vi "HEWH First Hour Rating Previous Terminate Value.vi"(8 "Error In":errorcluster, 11 "FileInit Cluster":T1={"Scan Rate Adjust"=0.0, "Draw Count"=0, "Test Patten Setup"={"Total Gallons Schedule"=[], "PRAT/RLT Sequence"=[{"Sequence #"=1.0, "Cycles"=35, "Mode Setting"="", "Flow Rate (GPM)"=0.0, "Temperature (F)"=0.0, "Reset Timer"=FALSE, "Use Temp Decline Method"=FALSE, "Terminate Condition"=enum."C1-Terminate Draw @ Gallon Mark", "Condition Value #1"=0.0, "UE"=FALSE, "LE"=FALSE, "Comp"=FALSE, "Fan"=FALSE, "Test End Time (Sec)"=0.0, "Purge Until Cutout"=FALSE, "Start Conditions"=enum."Heat Source Cutout", "Condition Value #2"=0.0, "Remove Power"=FALSE, "Time"=0.0, "Check Special Cond."=enum."SC1-Do Nothing", "Condition#"=enum."C1", "Draw Flags"=enum."N/A", "Data Processing Delay (FHD 15sec, UEF 5 Sec)"=0.0, "Test Complete"=FALSE}, {"Sequence #"=2.0, "Cycles"=15, "Mode Setting"="", "Flow Rate (GPM)"=0.0, "Temperature (F)"=0.0, "Reset Timer"=FALSE, "Use Temp Decline Method"=FALSE, "Terminate Condition"=enum."C1-Terminate Draw @ Gallon Mark", "Condition Value #1"=0.0, "UE"=FALSE, "LE"=FALSE, "Comp"=FALSE, "Fan"=FALSE, "Test End Time (Sec)"=0.0, "Purge Until Cutout"=FALSE, "Start Conditions"=enum."Heat Source Cutout", "Condition Value #2"=0.0, "Remove Power"=FALSE, "Time"=0.0, "Check Special Cond."=enum."SC1-Do Nothing", "Condition#"=enum."C1", "Draw Flags"=enum."N/A", "Data Processing Delay (FHD 15sec, UEF 5 Sec)"=0.0, "Test Complete"=FALSE}, {"Sequence #"=3.0, "Cycles"=35, "Mode Setting"="", "Flow Rate (GPM)"=0.0, "Temperature (F)"=0.0, "Reset Timer"=FALSE, "Use Temp Decline Method"=FALSE, "Terminate Condition"=enum."C1-Terminate Draw @ Gallon Mark", "Condition Value #1"=0.0, "UE"=FALSE, "LE"=FALSE, "Comp"=FALSE, "Fan"=FALSE, "Test End Time (Sec)"=0.0, "Purge Until Cutout"=FALSE, "Start Conditions"=enum."Heat Source Cutout", "Condition Value #2"=0.0, "Remove Power"=FALSE, "Time"=0.0, "Check Special Cond."=enum."SC1-Do Nothing", "Condition#"=enum."C1", "Draw Flags"=enum."N/A", "Data Processing Delay (FHD 15sec, UEF 5 Sec)"=0.0, "Test Complete"=FALSE}, {"Sequence #"=4.0, "Cycles"=15, "Mode Setting"="", "Flow Rate (GPM)"=0.0, "Temperature (F)"=0.0, "Reset Timer"=FALSE, "Use Temp Decline Method"=FALSE, "Terminate Condition"=enum."C1-Terminate Draw @ Gallon Mark", "Condition Value #1"=0.0, "UE"=FALSE, "LE"=FALSE, "Comp"=FALSE, "Fan"=FALSE, "Test End Time (Sec)"=0.0, "Purge Until Cutout"=FALSE, "Start Conditions"=enum."Heat Source Cutout", "Condition Value #2"=0.0, "Remove Power"=FALSE, "Time"=0.0, "Check Special Cond."=enum."SC1-Do Nothing", "Condition#"=enum."C1", "Draw Flags"=enum."N/A", "Data Processing Delay (FHD 15sec, UEF 5 Sec)"=0.0, "Test Complete"=FALSE}, {"Sequence #"=5.0, "Cycles"=35, "Mode Setting"="", "Flow Rate (GPM)"=0.0, "Temperature (F)"=0.0, "Reset Timer"=FALSE, "Use Temp Decline Method"=FALSE, "Terminate Condition"=enum."C1-Terminate Draw @ Gallon Mark", "Condition Value #1"=0.0, "UE"=FALSE, "LE"=FALSE, "Comp"=FALSE, "Fan"=FALSE, "Test End Time (Sec)"=0.0, "Purge Until Cutout"=FALSE, "Start Conditions"=enum."Heat Source Cutout", "Condition Value #2"=0.0, "Remove Power"=FALSE, "Time"=0.0, "Check Special Cond."=enum."SC1-Do Nothing", "Condition#"=enum."C1", "Draw Flags"=enum."N/A", "Data Processing Delay (FHD 15sec, UEF 5 Sec)"=0.0, "Test Complete"=FALSE}, {"Sequence #"=6.0, "Cycles"=15, "Mode Setting"="", "Flow Rate (GPM)"=0.0, "Temperature (F)"=0.0, "Reset Timer"=FALSE, "Use Temp Decline Method"=FALSE, "Terminate Condition"=enum."C1-Terminate Draw @ Gallon Mark", "Condition Value #1"=0.0, "UE"=FALSE, "LE"=FALSE, "Comp"=FALSE, "Fan"=FALSE, "Test End Time (Sec)"=0.0, "Purge Until Cutout"=FALSE, "Start Conditions"=enum."Heat Source Cutout", "Condition Value #2"=0.0, "Remove Power"=FALSE, "Time"=0.0, "Check Special Cond."=enum."SC1-Do Nothing", "Condition#"=enum."C1", "Draw Flags"=enum."N/A", "Data Processing Delay (FHD 15sec, UEF 5 Sec)"=0.0, "Test Complete"=FALSE}, {"Sequence #"=7.0, "Cycles"=35, "Mode Setting"="", "Flow Rate (GPM)"=0.0, "Temperature (F)"=0.0, "Reset Timer"=FALSE, "Use Temp Decline Method"=FALSE, "Terminate Condition"=enum."C1-Terminate Draw @ Gallon Mark", "Condition Value #1"=0.0, "UE"=FALSE, "LE"=FALSE, "Comp"=FALSE, "Fan"=FALSE, "Test End Time (Sec)"=0.0, "Purge Until Cutout"=FALSE, "Start Conditions"=enum."Heat Source Cutout", "Condition Value #2"=0.0, "Remove Power"=FALSE, "Time"=0.0, "Check Special Cond."=enum."SC1-Do Nothing", "Condition#"=enum."C1", "Draw Flags"=enum."N/A", "Data Processing Delay (FHD 15sec, UEF 5 Sec)"=0.0, "Test Complete"=FALSE}, {"Sequence #"=8.0, "Cycles"=15, "Mode Setting"="", "Flow Rate (GPM)"=0.0, "Temperature (F)"=0.0, "Reset Timer"=FALSE, "Use Temp Decline Method"=FALSE, "Terminate Condition"=enum."C1-Terminate Draw @ Gallon Mark", "Condition Value #1"=0.0, "UE"=FALSE, "LE"=FALSE, "Comp"=FALSE, "Fan"=FALSE, "Test End Time (Sec)"=0.0, "Purge Until Cutout"=FALSE, "Start Conditions"=enum."Heat Source Cutout", "Condition Value #2"=0.0, "Remove Power"=FALSE, "Time"=0.0, "Check Special Cond."=enum."SC1-Do Nothing", "Condition#"=enum."C1", "Draw Flags"=enum."N/A", "Data Processing Delay (FHD 15sec, UEF 5 Sec)"=0.0, "Test Complete"=FALSE}], "Current Sequence Index"=0}, "HEWH Specific DAQ"={"HEWH Data"={"HEWH Standard"={"Voltage (Volts)"=0.0, "Current (Amps)"=0.0, "Power (Watts)"=0.0, "WattHours (Wh)"=0.0, "TC Tree (AVG)"=0.0, "Flow Rate (GPM)"=0.0, "Gallons (Gal)"=0.0, "RTD Out (Deg F)"=0.0, "RTD In (Deg F)"=0.0, "RTD Amb (Deg F)"=0.0, "TC Down"=0.0, "UE Event Lead"=0, "LE Event Lead"=0, "TC Tree Array"=[]}, "PRAT"={"Power (Watts) A"=4192.0, "Power (Watts) B"=4192.0, "Power (Watts) C"=4192.0, "Power (Watts) D"=4192.0, "TC1"=0.0, "TC2"=0.0, "TC3"=0.0, "TC4"=0.0, "WattHours (Wh) A"=4192.0, "WattHours (Wh) B"=4192.0, "WattHours (Wh) C"=4192.0, "WattHours (Wh) D"=4192.0, "Ambient"=0.0, "Extra Temp"=0.0}, "Additional Power Data"={"Vthd"=236.2, "Frequency (Hz)"=236.2, "Apparent Power (VA)"=236.2, "Power Factor"=236.2, "Current Crest Factor"=236.2, "Voltage Crest Factor"=236.2, "Integration Time (sec)"=236.2}}, "Flow Valve % Open"=0.0, "Power State"={"UE"=FALSE, "LE"=FALSE, "COMP"=FALSE, "FANS"=FALSE}, "Power Analyzer"=enum."", "Flow Valve uA Output"=0, "Gallons Start (Gal)"=0.0}, "Test Output Data"={"PreDraw Data Table"=[], "Data Table"=[], "MW100 TC Headers"=[]}, "Calc and Calibration"={"Mean SD Var Max Min Array"=[], "Draw Statistics (DBL)"=[], "Calibration Coefficients DBL"=[], "Start Gallons"=0.0, "Starting Temp Decline"=0.0, "K-Factor (Intellifaucet)"=0.0, "All Draw Stats"=[], "RTD Terminate Value"=0.0}, "Current Draw Time"=0.0, "LV Program"=enum."HEWH", "Station ID"=enum."A", "Current Cond"=enum."N/A", "Test Complete"=FALSE} {"Test Patten Setup"."PRAT/RLT Sequence"."Time" format="%<%H:%M:%S>t"; "Test Patten Setup"."Total Gallons Schedule" format="%.2f"}) -> (0 "Error Out":errorcluster, 3 "Previous Terminate Value":dbl=115.0)   [LabVIEW 2016]
uses:
  Type Definitions/HEWH Output Information.ctl
  Type Definitions/HEWH Draw Pattern Setup.ctl
  Type Definitions/PRAT Test.ctl
  Utility/Save File/File Setup (Public)/Type Definition/Save File HEWH Heating Control Mode.ctl
  Draw Water Specific/Type Definitions/Terminate Draw Conditions.ctl
  Type Definitions/HEWH Start Conditions.ctl
  Draw Water Specific/Type Definitions/Check Special Condtions.ctl
  Draw Water Specific/Type Definitions/HEWH Special Condition Check.ctl
  Type Definitions/HEWH Draw Flag ENUM.ctl
  Type Definitions/HEWH Specific DAQ.ctl
  Type Definitions/HEWH Power Data.ctl
  Type Definitions/HEWH Power Elements.ctl
  Utility/Type Definitions/UTILITY Power Analyzer.ctl
  Type Definitions/HEWH Calc and Calibration.ctl
  Utility/Save File/File Setup (Public)/Type Definition/Save File DOE LabView Program.ctl
  Custom Instrument Control/MW100/Type Definitions/Station ID Selector.ctl
  <vilib>/Utility/file.llb/Read From Spreadsheet File (string).vi
  Utility/Save File/File Setup.lvlib
panel:
  out "all rows":string[][](array[string])
  in  "file path (dialog if empty)":path
  in  "Debug":string[][](array[string])=[["Voltage (Volts) - Mean", "Voltage (Volts) - Standard Deviation", "Voltage (Volts) - Variance", "Voltage (Volts) - Max", "Voltage (Volts) - Min", "Current (Amps) - Mean", "Current (Amps) - Standard Deviation", "Current (Amps) - Variance", "Current (Amps) - Max", "Current (Amps) - Min", "Power (Watts) - Mean", "Power (Watts) - Standard Deviation", "Power (Watts) - Variance", "Power (Watts) - Max", "Power (Watts) - Min", "WattHours - Max", "WattHours - Min", "TC Tree (AVG) - Mean", "TC Tree (AVG) - Standard Deviation", "TC Tree (AVG) - Variance", "TC Tree (AVG) - Max", "TC Tree (AVG) - Min", "Flow Rate (GPM) - Mean", "Flow Rate (GPM) - Standard Deviation", "Flow Rate (GPM) - Variance", "Flow Rate (GPM) - Max", "Flow Rate (GPM) - Min", "Gallons (Gal) - Max", "Gallons (Gal) - Min", "RTD Out (°F) - Mean", "RTD Out (°F) - Standard Deviation", "RTD Out (°F) - Variance", "RTD Out (°F) - Max", "RTD Out (°F) - Min", "RTD In (°F) - Mean", "RTD In (°F) - Standard Deviation", "RTD In (°F) - Variance", "RTD In (°F) - Max", "RTD In (°F) - Min", "RTD Ambinet (°F) - Mean", "RTD Ambient (°F) - Standard Deviation", "RTD Ambinent (°F) - Variance", "RTD Ambinent (°F) - Max", "RTD Ambinent (°F) - Min", "TC Down (°F) - Mean", "TC Down (°F) - Standard Deviation", "TC Down (°F) - Variance", "TC Down (°F) - Max", "TC Down (°F) - Min", "TC1 (°F) - Mean", "TC1 (°F) - Standard Deviation", "TC1 (°F) - Variance", "TC1 (°F) - Max", "TC1 (°F) - Min", "TC2 (°F) - Mean", "TC2 (°F) - Standard Deviation", "TC2 (°F) - Variance", "TC2 (°F) - Max", "TC2 (°F) - Min", "TC3 (°F) - Mean", "TC3 (°F) - Standard Deviation", "TC3 (°F) - Variance", "TC3 (°F) - Max", "TC3 (°F) - Min", "TC4 (°F) - Mean", "TC4 (°F) - Standard Deviation", "TC4 (°F) - Variance", "TC4 (°F) - Max", "TC4 (°F) - Min", "TC5 (°F) - Mean", "TC5 (°F) - Standard Deviation", "TC5 (°F) - Variance", "TC5 (°F) - Max", "TC5 (°F) - Min", "TC6 (°F) - Mean", "TC6 (°F) - Standard Deviation", "TC6 (°F) - Variance", "TC6 (°F) - Max", "TC6 (°F) - Min", "Total Harmonic Distortion (%V) - Max", "Total Harmonic Distortion (%V) - Min", "Frequency (Hz) - Mean ", "Frequency (Hz) - Standard Deviation", "Frequency (Hz) - Variance", "Frequency (Hz) - Max", "Frequency (Hz) - Min", "Apparent Power (VA) - Mean", "Apparent Power (VA) - Standard Deviation", "Apparent Power (VA) - Variance", "Apparent Power (VA) - Max", "Apparent Power (VA) - Min", "Power Factor - Max", "Power Factor - Min", "Current Crest Factor - Max", "Current Crest Factor - Min", "Voltage Crest Factor - Max", "Voltage Crest Factor - Min", "Elapsed Time (Sec) - Max", "Elapsed Time (Sec) - Min", "Condition Value #1", "Draw Count", ""], ["240.015", "0.427", "0.183", "240.270", "238.890", "0.378", "0.815", "0.665", "2.251", "0.014", "73.509", "164.034", "26907.243", "441.200", "1.055", "0.419", "0.077", "125.490", "0.253", "0.064", "125.800", "124.917", "3.018", "0.064", "0.004", "3.160", "2.900", "1.550", "0.830", "127.000", "0.000", "0.000", "127.000", "127.000", "57.575", "0.464", "0.215", "58.700", "57.000", "70.067", "0.048", "0.002", "70.100", "70.000", "57.929", "0.524", "0.274", "58.700", "57.200", "128.500", "0.000", "0.000", "128.500", "128.500", "128.312", "0.034", "0.001", "128.400", "128.300", "128.100", "0.000", "0.000", "128.100", "128.100", "127.700", "0.000", "0.000", "127.700", "127.700", "125.454", "1.114", "1.241", "126.200", "122.700", "114.875", "0.523", "0.273", "116.000", "114.200", "1.734", "1.563", "60.025", "0.015", "0.000", "60.063", "59.998", "90.320", "194.990", "38021.086", "539.800", "3.467", "0.856", "0.296", "9.576", "1.605", "1.449", "1.418", "29.823", "15.517", "0.000", "0.000", ""], ["239.536", "0.610", "0.372", "242.500", "238.460", "7.472", "8.359", "69.877", "18.776", "0.014", "1762.908", "2029.049", "4117040.569", "4510.000", "1.035", "597.580", "255.570", "104.807", "13.752", "189.114", "128.500", "82.400", "3.003", "0.059", "0.004", "3.170", "2.800", "33.840", "0.780", "127.270", "3.423", "11.719", "131.000", "116.000", "57.578", "0.360", "0.130", "58.900", "56.800", "69.441", "0.264", "0.070", "69.900", "68.800", "57.952", "0.451", "0.203", "59.200", "56.800", "126.863", "5.421", "29.387", "131.700", "105.800", "119.154", "17.250", "297.576", "131.600", "81.000", "107.909", "22.756", "517.820", "131.500", "78.000", "96.487", "20.170", "406.839", "130.600", "77.100", "89.568", "13.478", "181.656", "127.900", "75.200", "88.858", "12.000", "144.005", "117.700", "75.400", "1.682", "1.491", "59.995", "0.014", "0.000", "60.061", "59.946", "1794.387", "2009.288", "4037238.121", "4510.000", "3.430", "1.000", "0.291", "9.827", "1.421", "1.438", "1.418", "675.733", "15.038", "15.000", "0.000", ""]]
  in  "RTD Max Min Array":string[][](array[string])=[["", "", "", ""]]
  # "Draw Pattern Setup (24 Hour)"
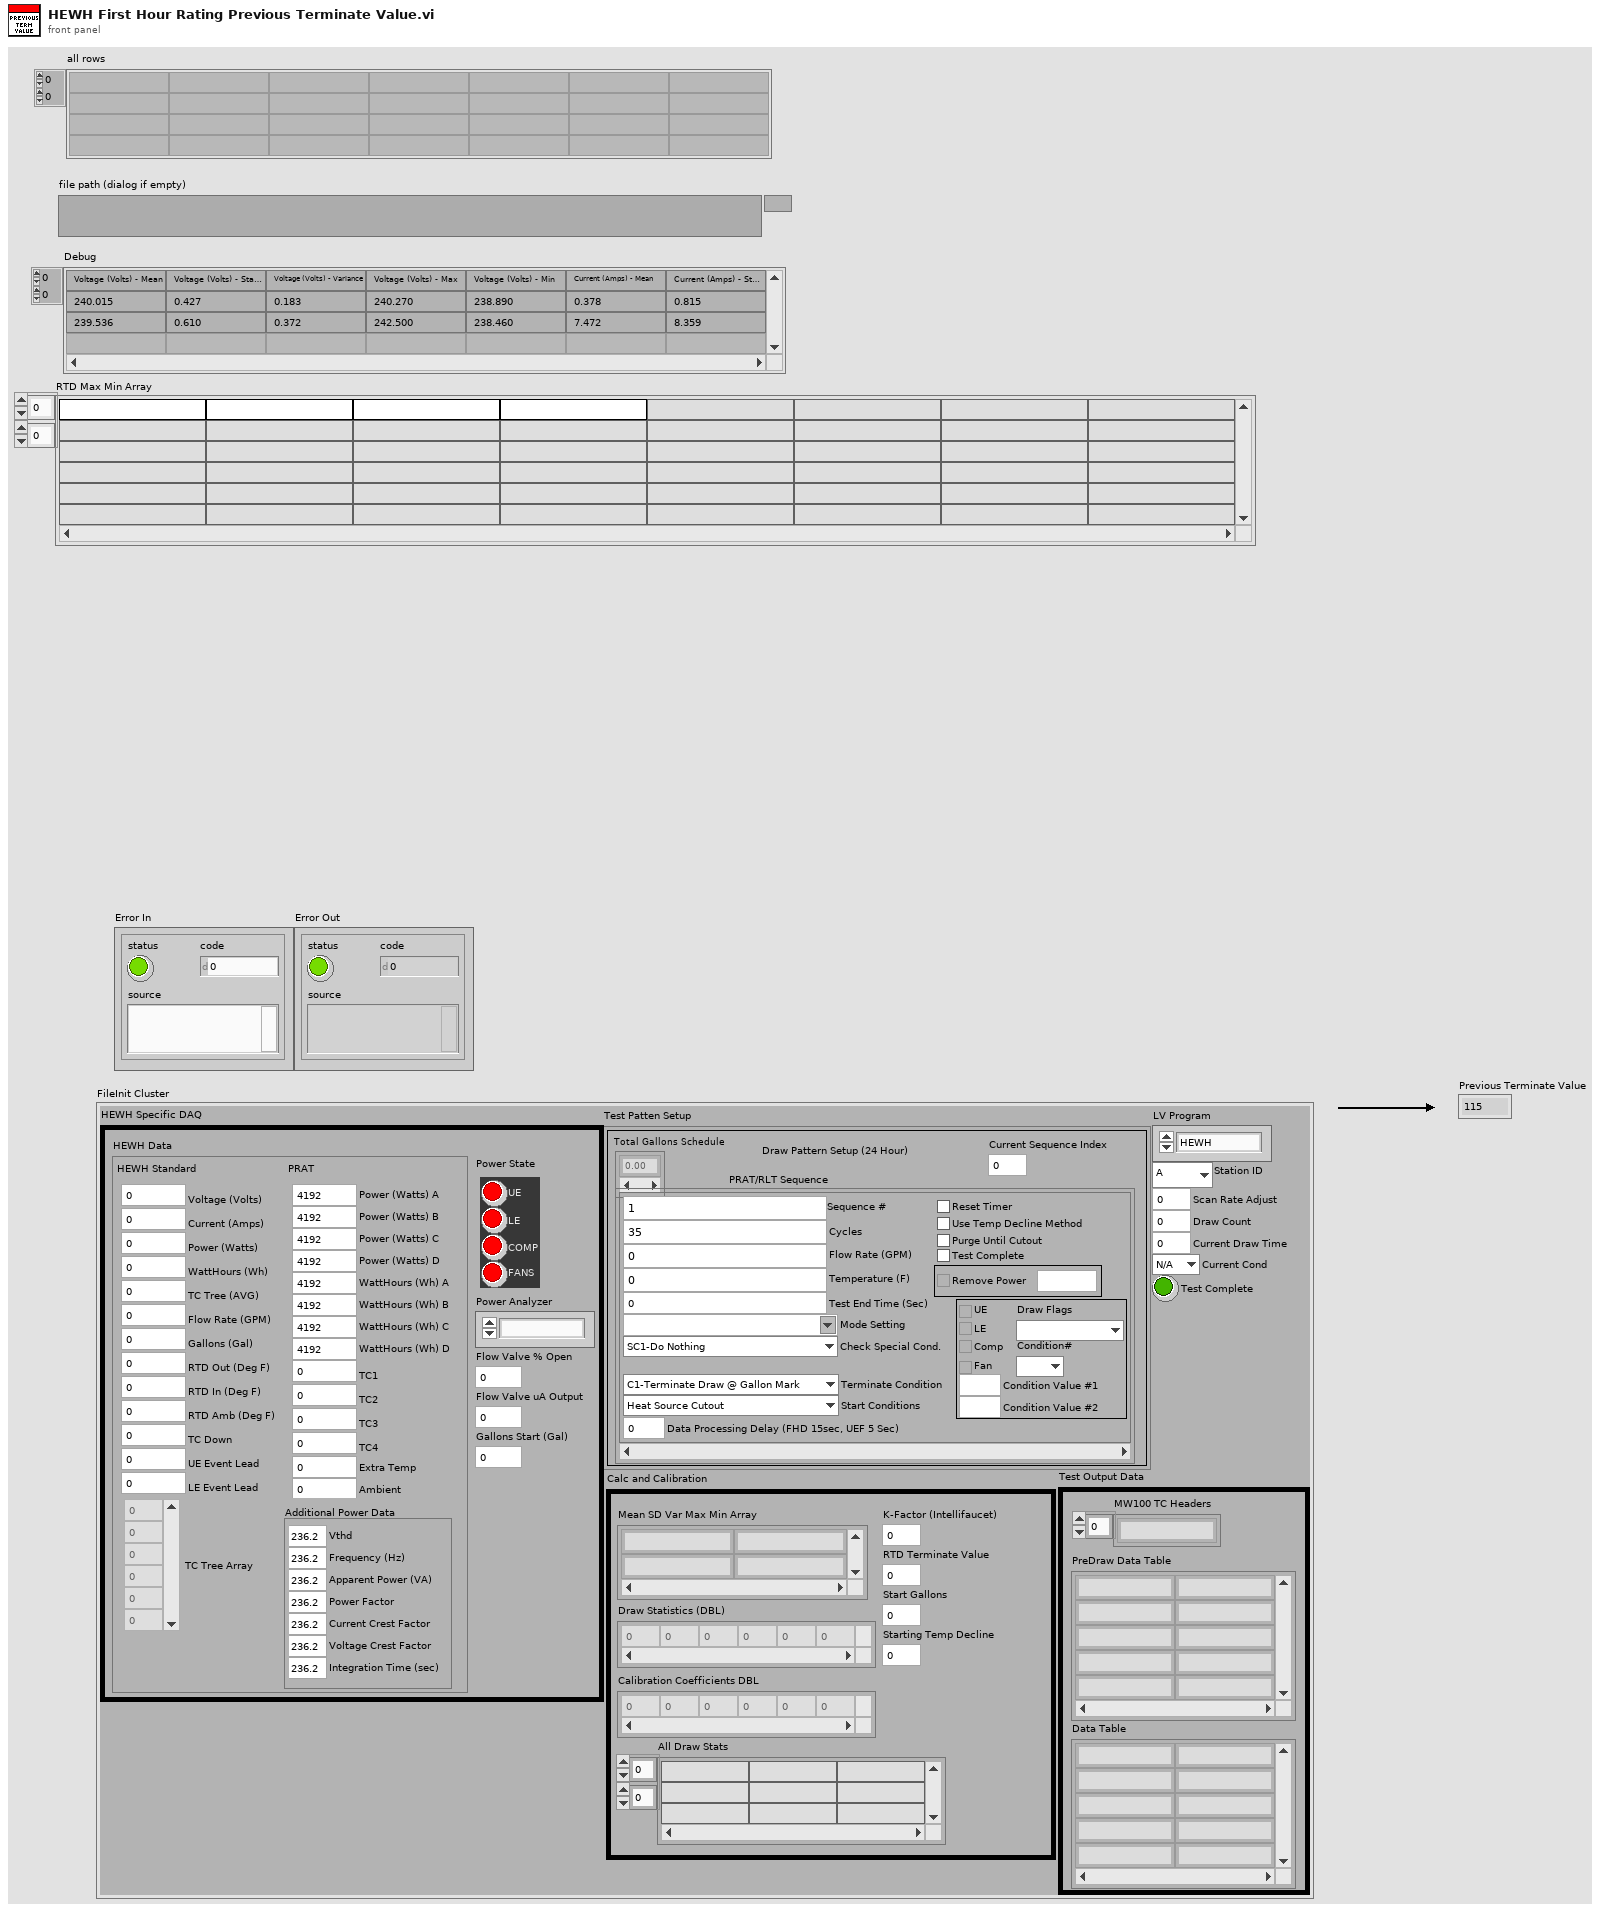
[diagram p1: front panel]
types:
  T1 = typedef "HEWH Output Information.ctl" = cluster{"Scan Rate Adjust":dbl, "Draw Count":i32, "Test Patten Setup":T2, "HEWH Specific DAQ":T10, "Test Output Data":cluster{"PreDraw Data Table":string[][], "Data Table":string[][], "MW100 TC Headers":string[]}, "Calc and Calibration":T14, "Current Draw Time":dbl, "LV Program":T15, "Station ID":T16, "Current Cond":T8, "Test Complete":bool}
  T2 = typedef "HEWH Draw Pattern Setup.ctl" = cluster{"Total Gallons Schedule":dbl[], "PRAT/RLT Sequence":T3[], "Current Sequence Index":i32}
  T3 = typedef "PRAT Test.ctl" = cluster{"Sequence #":dbl, "Cycles":i32, "Mode Setting":T4, "Flow Rate (GPM)":dbl, "Temperature (F)":dbl, "Reset Timer":bool, "Use Temp Decline Method":bool, "Terminate Condition":T5, "Condition Value #1":dbl, "UE":bool, "LE":bool, "Comp":bool, "Fan":bool, "Test End Time (Sec)":dbl, "Purge Until Cutout":bool, "Start Conditions":T6, "Condition Value #2":dbl, "Remove Power":bool, "Time":dbl, "Check Special Cond.":T7, "Condition#":T8, "Draw Flags":T9, "Data Processing Delay (FHD 15sec, UEF 5 Sec)":dbl, "Test Complete":bool}
  T4 = typedef "File Setup.lvlib/Save File HEWH Heating Control Mode.ctl" = string
  T5 = typedef "Terminate Draw Conditions.ctl" = enum16{"C1-Terminate Draw @ Gallon Mark", "C2-Special Last Draw (HU Test)", "C3-RTD Out <=", "C4-Mean Tank Temp <=", "C5-Decrease RTD Out (Deg F)", "C6-Time (Seconds)", "C7-Until Any Heat Source", "C8-Specific Heat Source", "C9-Do Nothing"}
  T6 = typedef "HEWH Start Conditions.ctl" = enum16{"Heat Source Cutout", "At Time (Seconds)", "Every X (Seconds)", "T2 >= X° Below Setpoint", "Seconds From Complete", "Wait for LE & Comp Cutout", "Wait for Comp Cutout", "Wait for LE Cutout", "Wait for UE Cutout"}
  T7 = typedef "Check Special Condtions.ctl" = enum16{"SC1-Do Nothing", "SC2-Check Heat Source (On-C2/Off-C1)", "SC3-Check Skip Condition", "SC4-Check Heat Source ON/Fail"}
  T8 = typedef "HEWH Special Condition Check.ctl" = enum16{"N/A", "C1", "C2", "Reset/Fail", "Skip Draw Sequence"}
  T9 = typedef "HEWH Draw Flag ENUM.ctl" = enum16{"N/A", "None(0)", "Sml(1)", "Med(2)", "SmlMed(3)", "Lrg(4)", "SmlLrg(5)", "MedLrg(6)", "SmlMedLrg(7)"}
  T10 = typedef "HEWH Specific DAQ.ctl" = cluster{"HEWH Data":T11, "Flow Valve % Open":dbl, "Power State":T12, "Power Analyzer":T13, "Flow Valve uA Output":i32, "Gallons Start (Gal)":dbl}
  T11 = typedef "HEWH Power Data.ctl" = cluster{"HEWH Standard":cluster{"Voltage (Volts)":dbl, "Current (Amps)":dbl, "Power (Watts)":dbl, "WattHours (Wh)":dbl, "TC Tree (AVG)":dbl, "Flow Rate (GPM)":dbl, "Gallons (Gal)":dbl, "RTD Out (Deg F)":dbl, "RTD In (Deg F)":dbl, "RTD Amb (Deg F)":dbl, "TC Down":dbl, "UE Event Lead":i32, "LE Event Lead":i32, "TC Tree Array":dbl[]}, "PRAT":cluster{"Power (Watts) A":dbl, "Power (Watts) B":dbl, "Power (Watts) C":dbl, "Power (Watts) D":dbl, "TC1":dbl, "TC2":dbl, "TC3":dbl, "TC4":dbl, "WattHours (Wh) A":dbl, "WattHours (Wh) B":dbl, "WattHours (Wh) C":dbl, "WattHours (Wh) D":dbl, "Ambient":dbl, "Extra Temp":dbl}, "Additional Power Data":cluster{"Vthd":dbl, "Frequency (Hz)":dbl, "Apparent Power (VA)":dbl, "Power Factor":dbl, "Current Crest Factor":dbl, "Voltage Crest Factor":dbl, "Integration Time (sec)":dbl}}
  T12 = typedef "HEWH Power Elements.ctl" = cluster{"UE":bool, "LE":bool, "COMP":bool, "FANS":bool}
  T13 = typedef "UTILITY Power Analyzer.ctl" = enum16{"", "APLUS", "WT210", "WT500", "WT300", "OSI", "Debug", "WT230", "WT300_1", "WT300_2"}
  T14 = typedef "HEWH Calc and Calibration.ctl" = cluster{"Mean SD Var Max Min Array":string[][], "Draw Statistics (DBL)":dbl[][], "Calibration Coefficients DBL":dbl[][], "Start Gallons":dbl, "Starting Temp Decline":dbl, "K-Factor (Intellifaucet)":dbl, "All Draw Stats":string[][], "RTD Terminate Value":dbl}
  T15 = typedef "File Setup.lvlib/Save File DOE LabView Program.ctl" = enum16{"No Name Found", "DOE Stand", "Dishwasher Kitchen", "Portable Stand", "HEWH", "Dryer", "Dryer WILT", "HCC", "PRAT", "HEWH RLT", "Refrigeration"}
  T16 = typedef "Station ID Selector.ctl" = enum16{"", "A", "B", "C", "D", "Global"}
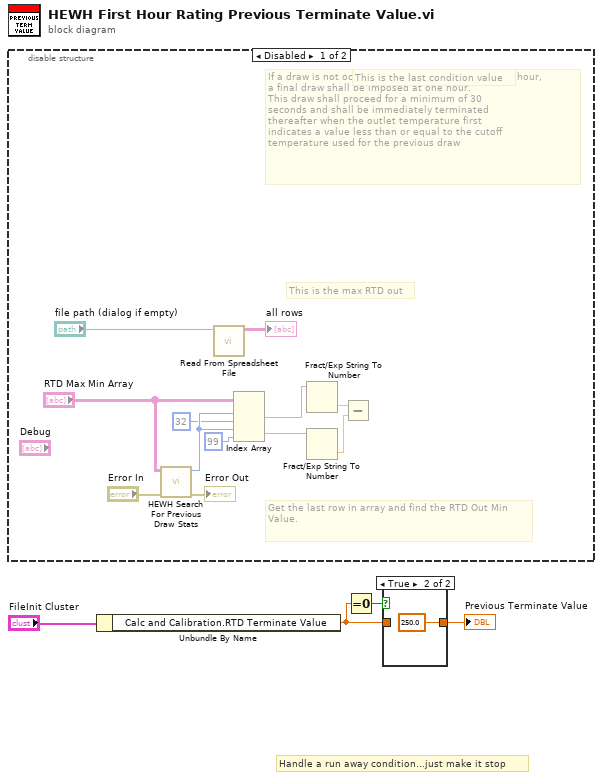
[diagram p0: block diagram]
diagram:
  # "Handle a run away condition...just make it stop"
  n1 = disable-structure shown="Disabled" {
    frame Disabled {
      # "This is the max RTD out"
      # "This is the last condition value"
      # "Get the last row in array and find the RTD Out Min\nValue."
      # "If a draw is not occurring at an elapsed time of one hour,\na final draw shall be imposed at one hour.\nThis draw shall proceed for a minimum of 30\nseconds and shall be immediately terminated\nthereafter when the outlet temperature first\nindicates a value less than or equal to the cutoff\ntemperature used for the previous draw"
      n2 = call "HEWH Search For Previous Draw Stats.vi"("Error In"="Error In", "RTD Max Min Array"="RTD Max Min Array") -> ("Error Out"=→"Error Out":errorcluster, "Previous Draw Stat Index (Row)"=w11:i32)  [unwired: 8 in]
      n3 = call-poly <vilib>:"Read From Spreadsheet File.vi"("file path (dialog if empty)"="file path (dialog if empty)") -> ("all rows"=→"all rows":string[][])  [unwired: 6 in, 4 out]
      n4 = Index Array(array="RTD Max Min Array", index (row) #1=w11, index (col) #1=32 ("disabled index (col)"), index (row) #2=w11, index (col) #2=99 ("disabled index (col)")) -> (element #1=w6:string, element #2=w8:string)
      n5 = Fract/Exp String To Number(string=w6) -> (number=w9:dbl)  [unwired: 3 in, 1 out]
      n6 = Fract/Exp String To Number(string=w8) -> (number=w10:dbl)  [unwired: 3 in, 1 out]
      n7 = Subtract(x=w9, y=w10) -> ()  [unwired: 1 out]
    }
    frame Enabled {
    }
  }
  n8 = Unbundle By Name("FileInit Cluster") -> ("Calc and Calibration.RTD Terminate Value"=w1:dbl)
  n9 = Equal To 0?(x=w1) -> (x = 0?=w3:bool)
  n10 = case shown="True" w3 {
    tunnel: [w17 250.0] -> w2
    tunnel: w1 -> [w17 _]
    frame False {
    }
    frame True {
    }
  }
  "Previous Terminate Value" <- w2
